vi "Process Return Value.vi"(8 "Error In":errorcluster, 10 "Proto Method VI":refnum<vi>, 11 "Simple Struct Writer in":refnum<class "Simple Struct Writer.lvclass">) -> (0 "Error Out":errorcluster, 1 "RetVal Param Info":T1={"Parameter Name"="", "Num Dimensions"=1, "Parameter Type"=enum."Numeric", "Numeric Type"=enum."I32", "Param Passing"=enum."By Value", "Array Passing"=enum."Array Data Pointer", "String Passing"=enum."C String Pointer", "Adapt Format"=enum."By Value", "ActiveX Types"=enum."ActiveX Variant Pointer", "Const (unused)"=FALSE, "Minimum Size"=""}, 2 "Modified Proto Method  VI":refnum<vi>, 3 "Simple Struct Writer out":refnum<class "Simple Struct Writer.lvclass">)   [LabVIEW 2013, in "Simple Struct Writer.lvclass"]
uses:
  Simple Struct Writer.lvclass
  Data Structures/DLL Parameter Info.ctl
  Simple Struct Writer.lvclass/Simple Struct Writer.ctl
  Abstract Param Writer/Abstract Param Writer.lvclass
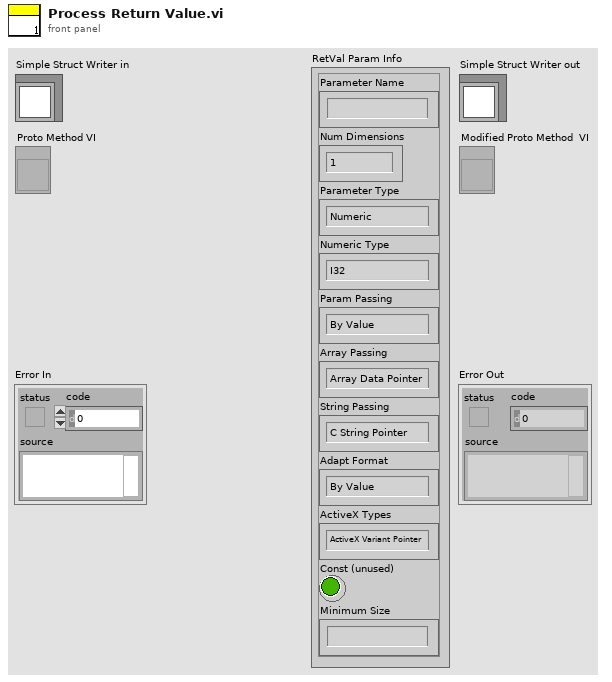
[diagram p1: front panel]
types:
  T1 = typedef "DLL Parameter Info.ctl" = cluster{"Parameter Name":string, "Num Dimensions":i32, "Parameter Type":enum16{"Numeric", "Array", "String", "Waveform", "Digital Waveform", "Digital Table", "ActiveX", "Any", "Instance Data Pointer", "Void"}, "Numeric Type":enum16{"I8", "I16", "I32", "I64", "U8", "U16", "U32", "U64", "SGL", "DBL", "PTR INT", "PTR UINT"}, "Param Passing":enum16{"By Value", "Pointer To Value"}, "Array Passing":enum16{"Array Data Pointer", "Array Handle", "Array Handle Pointer"}, "String Passing":enum16{"C String Pointer", "Pascal String Pointer", "String Handle", "String Handle Pointer"}, "Adapt Format":enum16{"By Value", "Pointer To Value"}, "ActiveX Types":enum16{"ActiveX Variant Pointer", "IDispatch* Pointer", "IUnknown* Pointer"}, "Const (unused)":bool, "Minimum Size":string}
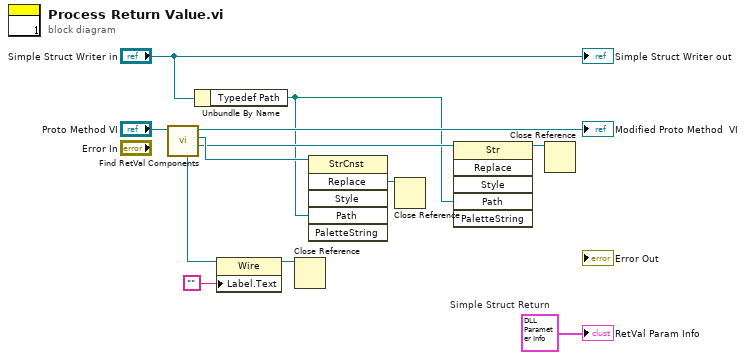
[diagram p0: block diagram]
diagram:
  w1 = T1 {"Parameter Name"="retVal", "Num Dimensions"=1, "Parameter Type"=enum."Any", "Numeric Type"=enum."I32", "Param Passing"=enum."By Value", "Array Passing"=enum."Array Data Pointer", "String Passing"=enum."C String Pointer", "Adapt Format"=enum."Pointer To Value", "ActiveX Types"=enum."ActiveX Variant Pointer", "Const (unused)"=FALSE, "Minimum Size"=""}  # Simple Struct Return
  n1 = call "Find RetVal Components.vi"("Proto Method VI"="Proto Method VI") -> ("Indicator"=w4:refnum<vi>, "Data Buffer"=w6:refnum<vi>, "Proto Method VI Dup"=→"Modified Proto Method  VI":refnum<vi>, "Wire"=w9:refnum<vi>)  [unwired: 6 in, 1 out]
  n2 = Unbundle By Name("Simple Struct Writer in") -> ("Typedef Path"=w3:path)
  n3 = property class="Wire"(reference=w9, "Label.Text"="") -> (reference out=w8:refnum<vi>)  [unwired: 1 in, 1 out]
  n4 = Close Reference(reference=w8) -> ()  [unwired: 1 in, 1 out]
  n5 = invoke class="StrCnst" method="Replace"(reference=w6, "Path"=w3) -> ("Replace"=w5:refnum<vi>)  [unwired: 4 in, 5 out]
  n6 = Close Reference(reference=w5) -> ()  [unwired: 1 in, 1 out]
  n7 = invoke class="Str" method="Replace"(reference=w4, "Path"=w3) -> (reference out=w2:refnum<vi>)  [unwired: 4 in, 5 out]
  n8 = Close Reference(reference=w2) -> ()  [unwired: 1 in, 1 out]
  "Simple Struct Writer out" <- "Simple Struct Writer in"
  "RetVal Param Info" <- w1
